vi "GenTrajFromMatlab.vi"() -> (1 "D3":dbl[](graph), 2 "Theta 2":dbl[](graph), 3 "Theta 1":dbl[](graph))   [LabVIEW 2016]
panel:
  out "Indexed XYZ Posit":dbl[](array[numeric])
  in  "Trajectory Type":enum16{"Vertical", "Parabolic", "Raster Scan"}(ring)=enum."Parabolic"
  in  "Ts":dbl=0.001
  out "Joint Arrays":dbl[][](array[numeric])
  out "Z":dbl[](graph)
  out "Y":dbl[](graph)
  out "X":dbl[](graph)
  in  "Speed [mm/s]":dbl=2.0
  in  "No Cycle":dbl=1.0
  in  "Travel":dbl=8.0 format="%#_13g"
  in  "Curvature":dbl=0.1
  in  "Origin Offset":dbl[](array[numeric])=[0.0, 4.0, -4.0]
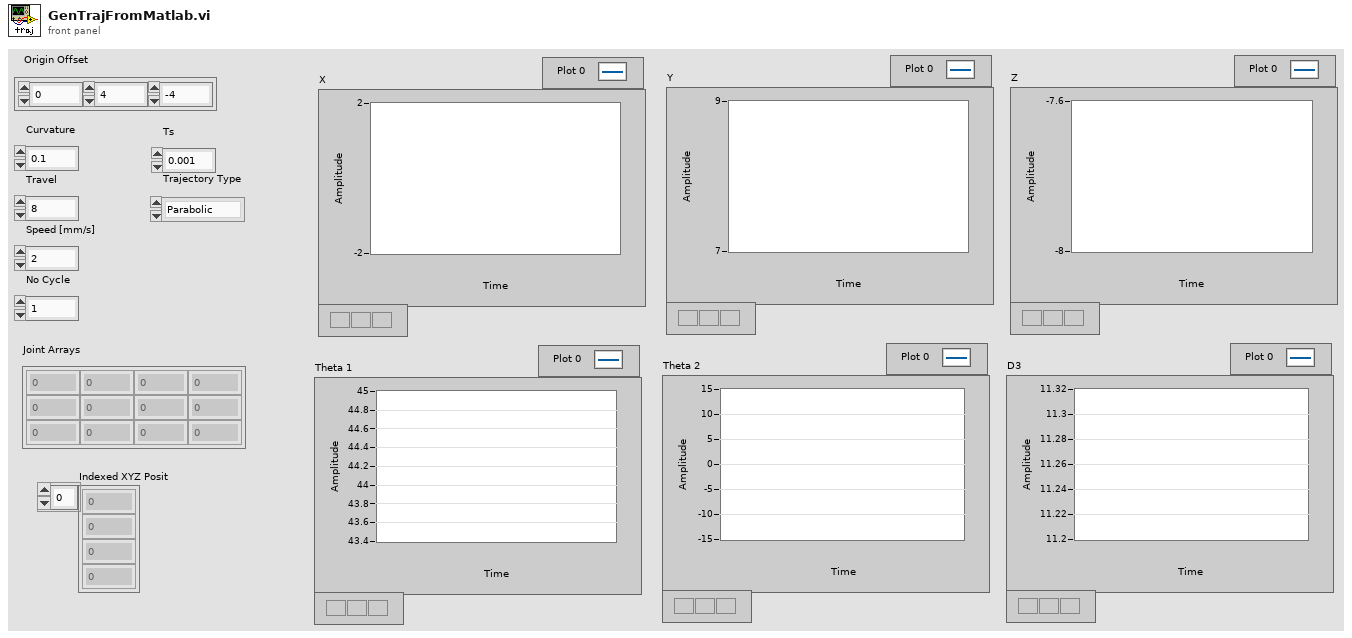
[diagram p1: front panel]
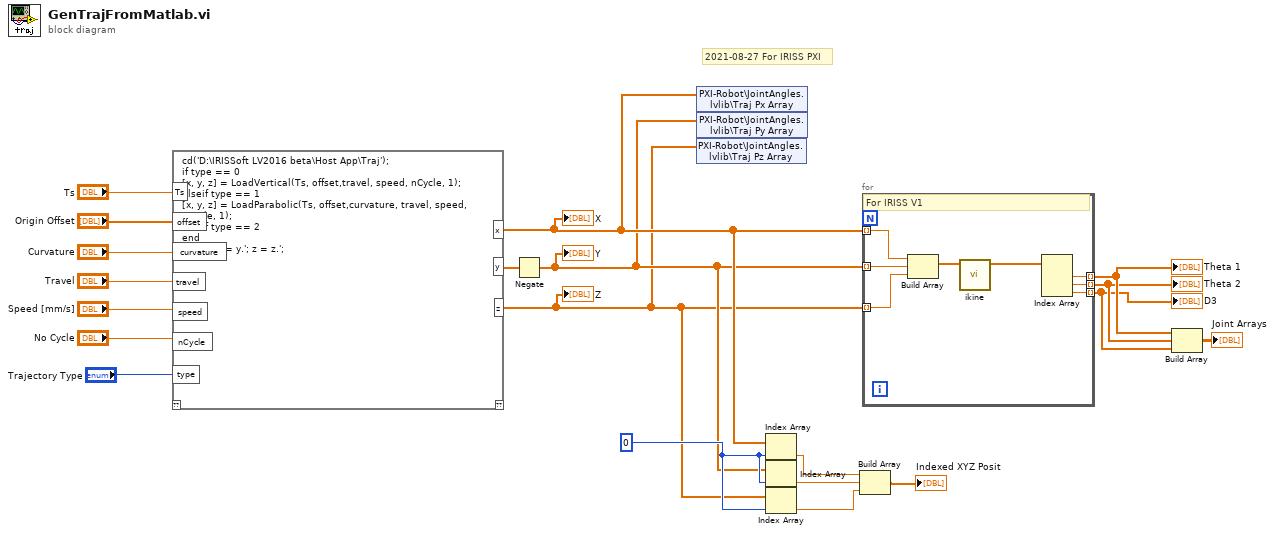
[diagram p0: block diagram]
diagram:
  w9 = 0 ("index")
  # "2021-08-27 For IRISS PXI"
  n1 = script code="cd('D:\\IRISSoft LV2016 beta\\Host App\\Traj');\nif type == 0\n[x, y, z] = LoadVertical(Ts, offset,travel, speed, nCycle, 1);\nelseif type == 1\n[x, y, z] = LoadParabolic(Ts, offset,curvature, travel, speed, nCycle, 1);\nelseif type == 2\nend\nx = x.'; y = y.'; z = z.';"("Ts"="Ts", "offset"="Origin Offset", "curvature"="Curvature", "travel"="Travel", "nCycle"="No Cycle", "speed"="Speed [mm/s]", "type"="Trajectory Type") -> ("x"=w3:dbl[], "y"=w4:dbl[], "z"=w1:dbl[])  [unwired: 1 in, 1 out]
  "X" <- w3
  "Z" <- w1
  n2 = Negate(x=w4) -> (-x=w2:dbl[])
  "Y" <- w2
  n3 = shared-variable "PXI-Robot\\JointAngles.lvlib\\Traj Px Array"(w3) -> ()  [unwired: 1 in, 1 out]
  n4 = shared-variable "PXI-Robot\\JointAngles.lvlib\\Traj Py Array"(w2) -> ()  [unwired: 1 in, 1 out]
  n5 = shared-variable "PXI-Robot\\JointAngles.lvlib\\Traj Pz Array"(w1) -> ()  [unwired: 1 in, 1 out]
  n6 = Index Array(array=w3, index=w9) -> (element=w8:dbl)
  n7 = Index Array(array=w2, index=w9) -> (element=w7:dbl)
  n8 = Index Array(array=w1, index=w9) -> (element=w6:dbl)
  n9 = Build Array(w8, w7, w6) -> (→"Indexed XYZ Posit":dbl[])
  n10 = for {
    tunnel: w3 -> [w28] mode=indexing
    tunnel: w2 -> [w26] mode=indexing
    tunnel: w1 -> [w25] mode=indexing
    tunnel: [w24] -> w15 mode=indexing
    tunnel: [w23] -> w14 mode=indexing
    tunnel: [w22] -> w13 mode=indexing
    # "For IRISS V1"
    n11 = Build Array(w28, w26, w25) -> (w27:dbl[])
    n12 = call "ikine.vi"("Tip XYZ Posit [mm]"=w27) -> ("Joint Posit [deg,deg,mm]"=w21:dbl[])  [unwired: 10 in]
    n13 = Index Array(array=w21) -> (element #1=w24:dbl, element #2=w23:dbl, element #3=w22:dbl)  [unwired: 3 in]
  }
  "Theta 1" <- w15
  "Theta 2" <- w14
  "D3" <- w13
  n14 = Build Array(w15, w14, w13) -> (→"Joint Arrays":dbl[][])
